vi "myRIO_BRig_RT_dataExp_ENL_penalty.vi"() -> (2 "output_ENL_penalty":i32)   [LabVIEW 2014]
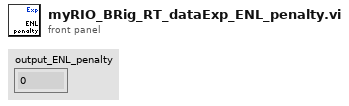
[diagram p1: front panel]
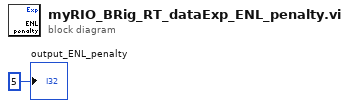
[diagram p0: block diagram]
diagram:
  "output_ENL_penalty" <- 5 ("output_iBlock")
